vi "Idle_WeatherStationMakePlots.vi"(4 "Weather Station Parsed List":string[](array[string])=["DAQ Settings", "Laser Control", "Real Time Charts", "Polarization Control", "Other ", "", "Endline"]) -> (0 "Ab/ Rel Humidity":dbl[][](graph), 1 "Weather StationData":dbl[][](graph), 2 "Temp/Press":dbl[][](graph), 3 "(X and Y arrays) Multi Plot":cluster{dbl[], dbl[]}[](graph), 5 "WeatherStationData":T1)   [LabVIEW 2012]
uses:
  WVDIAL_GlobalVariables.vi
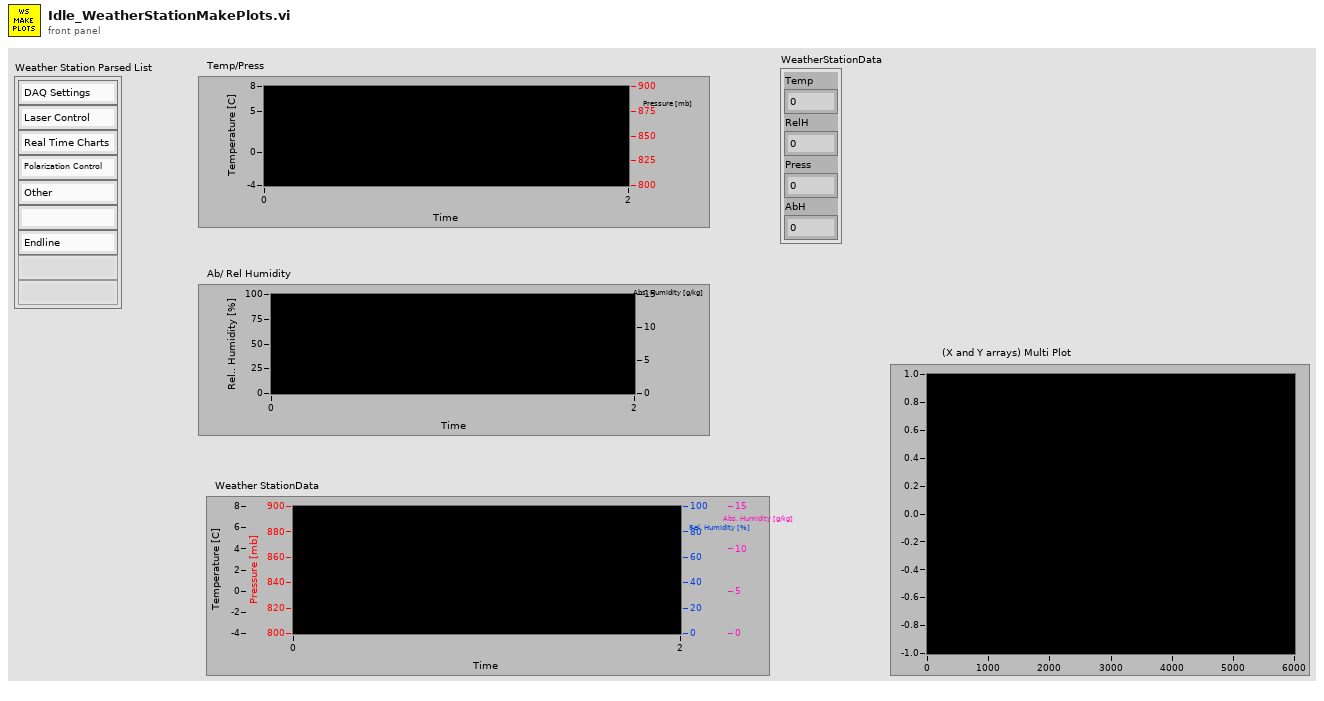
[diagram p1: front panel]
types:
  T1 = cluster{"Temp":dbl, "RelH":dbl, "Press":dbl, "AbH":dbl}
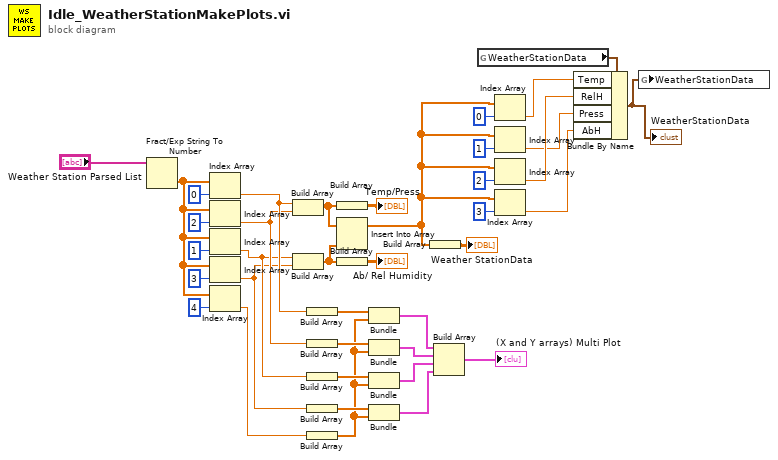
[diagram p0: block diagram]
diagram:
  n1 = Fract/Exp String To Number(string="Weather Station Parsed List") -> (number=w13:dbl[])  [unwired: 3 in, 1 out]
  n2 = Index Array(array=w13, index=0) -> (element=w8:dbl)
  n3 = Index Array(array=w13, index=2) -> (element=w7:dbl)
  n4 = Index Array(array=w13, index=1) -> (element=w6:dbl)
  n5 = Index Array(array=w13, index=3) -> (element=w5:dbl)
  n6 = Index Array(array=w13, index=4) -> (element=w4:dbl)
  n7 = Build Array(w8, w7) -> (w22:dbl[])
  n8 = Build Array(w6, w5) -> (w21:dbl[])
  n9 = Build Array(w8) -> (w10:dbl[])
  n10 = Build Array(w7) -> (w9:dbl[])
  n11 = Build Array(w6) -> (w3:dbl[])
  n12 = Build Array(w5) -> (w2:dbl[])
  n13 = Build Array(w4) -> (w1:dbl[])
  n14 = Build Array(w22) -> (→"Temp/Press":dbl[][])
  n15 = Insert Into Array(array=w22, new element=w21) -> (w18:dbl[])  [unwired: 1 in]
  n16 = Build Array(w21) -> (→"Ab/ Rel Humidity":dbl[][])
  n17 = Bundle "Bundle"(w10, w1) -> (w16:cluster{dbl[], dbl[]})  [unwired: 1 in]
  n18 = Bundle "Bundle"(w9, w1) -> (w17:cluster{dbl[], dbl[]})  [unwired: 1 in]
  n19 = Bundle "Bundle"(w3, w1) -> (w12:cluster{dbl[], dbl[]})  [unwired: 1 in]
  n20 = Bundle "Bundle"(w2, w1) -> (w11:cluster{dbl[], dbl[]})  [unwired: 1 in]
  n21 = Build Array(w18) -> (→"Weather StationData":dbl[][])
  n22 = Build Array "Build Array"(w16, w17, w12, w11) -> (→"(X and Y arrays) Multi Plot":cluster{dbl[], dbl[]}[])
  n23 = global read "WVDIAL_GlobalVariables.vi" "WeatherStationData"() -> (w25:T1)
  n24 = Index Array(array=w18, index=0) -> (element=w30:dbl)
  n25 = Index Array(array=w18, index=1) -> (element=w32:dbl)
  n26 = Index Array(array=w18, index=2) -> (element=w33:dbl)
  n27 = Index Array(array=w18, index=3) -> (element=w31:dbl)
  n28 = Bundle By Name(cluster=w25, "Temp"=w30, "RelH"=w33, "Press"=w32, "AbH"=w31) -> (w24:T1)
  "WeatherStationData" <- w24
  n29 = global write "WVDIAL_GlobalVariables.vi" "WeatherStationData"(w24) -> ()
